vi "reserve resource from client.vi"(7 "notes":string, 8 "error in (no error)":errorcluster, 9 "Name in Bitfile":string, 10 "Server Ref in":T1 format="%.0x", 11 "Item Ref in":T1 format="%.0x") -> (0 "error out":errorcluster, 3 "Item Ref out":T1 format="%.0x")   [LabVIEW 2016, in "FPGA RM Client API.lvlib"]
uses:
  FPGA RM Client API.lvlib
  <vilib>/NI Veristand/Custom Device API/Custom Device Item Ref.ctl
  <vilib>/NI VeriStand/Custom Device API/Custom Device API.lvlib
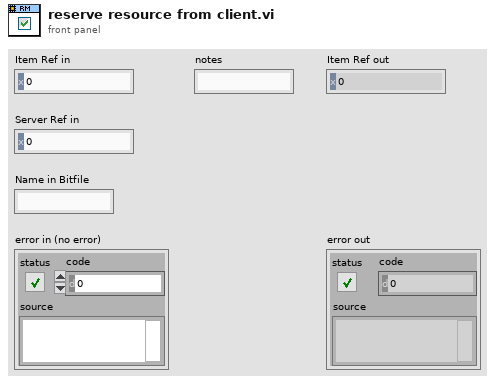
[diagram p1: front panel]
types:
  T1 = typedef "Custom Device API.lvlib/Custom Device Item Ref.ctl" = u64
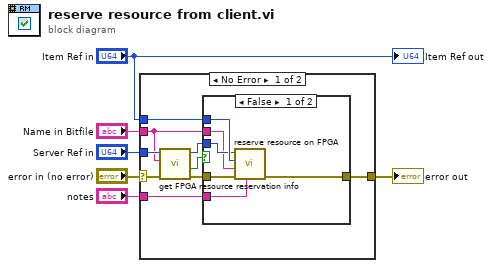
[diagram p0: block diagram]
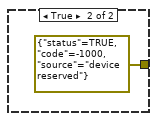
[diagram p2: hidden frame]
diagram:
  n1 = case shown="No Error" "error in (no error)" {
    selector: "error in (no error)" -> [w8 w23]
    tunnel: [w13 w23] -> w5
    tunnel: "Item Ref in" -> [w14 _]
    tunnel: "Server Ref in" -> [w12 _]
    tunnel: "notes" -> [w15 _]
    tunnel: "Name in Bitfile" -> [w10 _]
    frame No Error {
      n2 = call "get FPGA resource reservation info.vi"("error in (no error)"=w8, "Name in Bitfile"=w10, "Item Ref in"=w12) -> ("error out"=w7:errorcluster, "found?"=w9:bool, "Item Ref out"=w11:T1)  [unwired: 4 in, 2 out]
      n3 = case shown="False" w9 {
        tunnel: w15 -> [w16 _]
        tunnel: w14 -> [w21 _]
        tunnel: w7 -> [w20 _]
        tunnel: [w19 errorcluster {"status"=TRUE, "code"=-1000, "source"="device reserved"} ("error out")] -> w13
        tunnel: w11 -> [w18 _]
        tunnel: w10 -> [w17 _]
        frame False {
          n4 = call "reserve resource on FPGA.vi"("notes"=w16, "error in (no error)"=w20, "Name in bitfile"=w17, "Client Node Ref"=w21, "Item Ref in"=w18) -> ("error out"=w19:errorcluster)  [unwired: 5 in, 1 out]
        }
        frame True {
        }
      }
    }
    frame Error {
    }
  }
  "error out" <- w5
  "Item Ref out" <- "Item Ref in"
